vi "Plugin.Rx.Inline.Wait.vi"(8 "error in (no error)":errorcluster, 11 "Plugin in":refnum<class "Plugin.lvclass">) -> (0 "error out":errorcluster, 3 "Plugin out":refnum<class "Plugin.lvclass">)   [LabVIEW 2017, in "DSF Core.lvlib" / "Plugin.lvclass"]
uses:
  Plugin.lvclass
  Plugin.lvclass/Plugin.ctl
  Transfer/Transfer Group.lvclass/Transfer Group.ctl
  Timing/Timing.lvclass/Timing.ctl
  Debug/Debug Flags.lvclass/Debug Flags.ctl
  Debug/FIFO Flags.lvclass/FIFO Flags.ctl
  Transfer/Transfer.lvclass/Transfer.ctl
  <vilib>/NI/Memory Manager/Classes/Pointer/Memory.Pointer.lvclass/Memory.Pointer.ctl
  Transfer/Transfer Group.Return FIFO.Read.vi
  Transfer/Transfer Group.Get Transfers.vi
  Transfer/Transfer.Get Inline Buffer.vi
  Transfer/Transfer.Get Intermediate Buffer.vi
  <vilib>/NI/Memory Manager/Classes/Pointer/Memory.Pointer.Copy All.vi
  Transfer/Transfer Group.Get Return FIFO.vi
  Transfer/Transfer Group.Get Debug Flags.vi
  Debug/Debug Flags.Get FIFO Flags.vi
  Debug/FIFO Flags.Get Infinite Timeouts.vi
  <vilib>/NI/Memory Manager/Classes/Pointer/Memory.Pointer.Get Size.vi
  <vilib>/NI/Memory Manager/Classes/Pointer/Memory.Pointer.Copy.vi
  <vilib>/NI/Memory Manager/Classes/Pointer/Memory.Pointer.Copy.No Check.vi
  <vilib>/NI/Memory Manager/Classes/Pointer/Memory.Pointer.Parameter Check.Subset.vi
  <vilib>/NI/Memory Manager/Classes/Pointer/Memory.Pointer.Parameter Check.Null Pointer.vi
  <vilib>/NI/Memory Manager/Classes/Pointer/Memory.Pointer.Get Address.vi
  <vilib>/NI/Memory Manager/Classes/Pointer/Memory.Pointer.Errors.vi
  <vilib>/NI/Memory Manager/Classes/Pointer/Memory.Pointer.Errors.Out of Bounds.vi
  <vilib>/NI/Memory Manager/Classes/Pointer/Memory.Pointer.Errors.Null Pointer.vi
  <vilib>/NI/Memory Manager/VIs/Source.Write.String.vi
  <vilib>/NI/Memory Manager/Classes/Pointer/Memory.Pointer.Errors.Write Pointer Size.vi
  <vilib>/NI/Memory Manager/Classes/Pointer/Memory.Pointer.Errors.Create Error.vi
  <vilib>/NI/Memory Manager/VIs/Source.Write.Scalar.Base10.vi
  <vilib>/NI/Memory Manager/VIs/Source.Write.Scalar.Base10 (U64).vi
  <vilib>/NI/Memory Manager/VIs/New Error Cluster Constant.vi
  <vilib>/NI/Memory Manager/VIs/New Error Cluster Constant (512B).vi
  <vilib>/NI/Memory Manager/VIs/Error Cluster.Set Status.vi
  <vilib>/NI/Memory Manager/VIs/Error Cluster.Set Code.vi
  <vilib>/NI/Memory Manager/VIs/Error Cluster.Set VI Source.vi
  <vilib>/NI/Memory Manager/Constants/Memory.Constants.vi
  <vilib>/NI/Memory Manager/Constants/Memory.Constants.Library Name.vi
  <vilib>/NI/Memory Manager/Classes/Pointer/Memory.Pointer.Errors.Get Info.vi
  Pointer/DBL Pointer.lvclass
  C:/Program Files (x86)/National Instruments/LabVIEW 2017/vi.lib/NI/Memory Manager/Classes/Pointer/Memory.Pointer.lvclass
  Transfer/Transfer Group.Errors.vi
  Transfer/Transfer Group.Errors.Return Timeout.vi
  Transfer/Transfer Group.lvclass
  Timing/Timing.lvclass
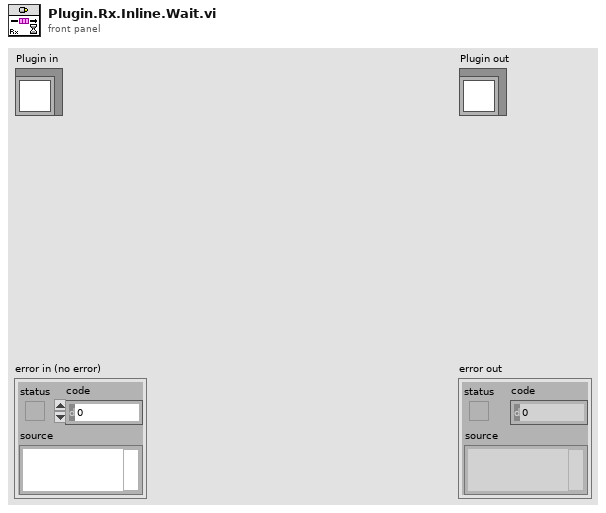
[diagram p1: front panel]
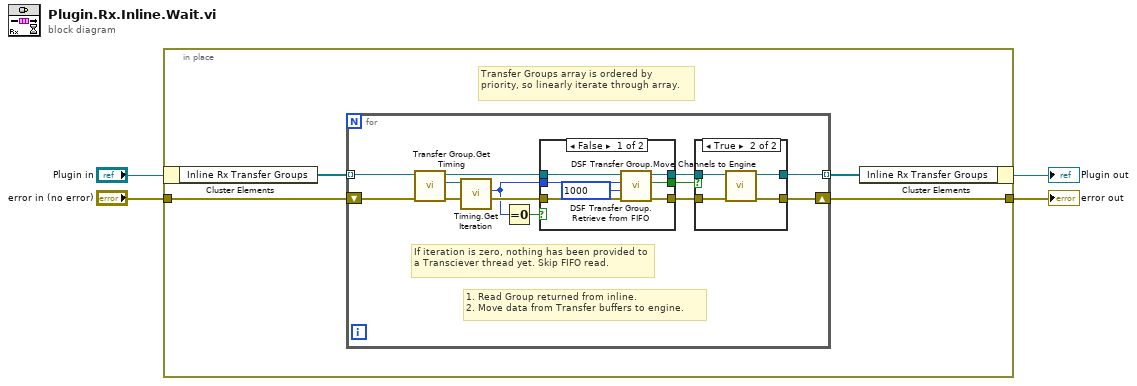
[diagram p0: block diagram]
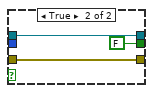
[diagram p3: hidden frame]
diagram:
  n1 = in-place {
    in-place-border: "error in (no error)" -> [w8]
    in-place-border: [w7] -> w4
    # "Transfer Groups array is ordered by priority, so linearly iterate through array."
    n2 = in-place-cluster #1("Plugin in") -> ("Inline Rx Transfer Groups"=w6:refnum<class "Transfer Group.lvclass">[])
    n3 = for {
      tunnel: w6 -> [w16] mode=indexing
      shift-right: [w10] -> w7
      shift-left: w8 -> [w15]
      tunnel: [w12] -> w5 mode=indexing
      # "If iteration is zero, nothing has been provided to a Transciever thread yet. Skip FIFO read."
      # "1. Read Group returned from inline.\n2. Move data from Transfer buffers to engine."
      n4 = call "Transfer Group.Get Timing.vi"("Transfer Group in"=w16) -> ("Timing"=w18:refnum<class "Timing.lvclass">, "Transfer Group out"=w17:refnum<class "Transfer Group.lvclass">)  [unwired: 9 in]
      n5 = call "Timing.Get Iteration.vi"("Timing in"=w18) -> ("Iteration"=w9:u64)  [unwired: 9 in, 1 out]
      n6 = Equal To 0?(x=w9) -> (x = 0?=w19:bool)
      n7 = case shown="False" w19 {
        tunnel: [w32 w35] -> w13
        tunnel: [w31 w33] -> w11
        tunnel: w17 -> [w30 w35]
        tunnel: w9 -> [w29 _]
        tunnel: [w28 FALSE ("iteration valid?")] -> w14
        tunnel: w15 -> [w26 w33]
        frame False {
          n8 = call "DSF Transfer Group.Retrieve from FIFO.vi"("error in (no error)"=w26, "timeout in ms (0)"=1000, "expected iteration"=w29, "Transfer Group in"=w30) -> ("error out"=w31:errorcluster, "iteration valid?"=w28:bool, "Transfer Group out"=w32:refnum<class "Transfer Group.lvclass">)  [unwired: 5 in]
        }
        frame True {
        }
      }
      n9 = case shown="True" w14 {
        tunnel: w13 -> [w21 w25]
        tunnel: [w21 w24] -> w12
        tunnel: w11 -> [w20 w23]
        tunnel: [w20 w22] -> w10
        frame False {
        }
        frame True {
          n10 = call "DSF Transfer Group.Move Channels to Engine.vi"("error in (no error)"=w23, "Transfer Group in"=w25) -> ("error out"=w22:errorcluster, "Transfer Group out"=w24:refnum<class "Transfer Group.lvclass">)  [unwired: 8 in]
        }
      }
    }
    n11 = in-place-cluster #1("Inline Rx Transfer Groups"=w5) -> (→"Plugin out":refnum<class "Plugin.lvclass">)
  }
  "error out" <- w4
